vi "vavle GELE.vi"(10 "output":dbl) -> (2 "T=Opening":bool)   [LabVIEW 2025]
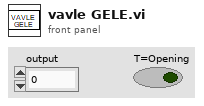
[diagram p1: front panel]
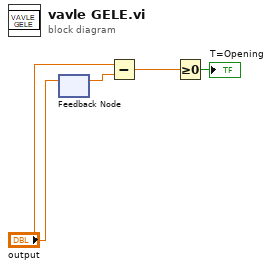
[diagram p0: block diagram]
diagram:
  n1 = feedback #1() -> (w1:dbl)  [unwired: 1 in]
  n2 = feedback-in #1("output") -> ()
  n3 = Subtract(x="output", y=w1) -> (x-y=w2:dbl)
  n4 = Greater Or Equal To 0?(x=w2) -> (x >= 0?=→"T=Opening":bool)
